vi "Create File Save Setup.vi"(8 "error in (no error)":errorcluster, 11 "Scan Data Process in":T1) -> (0 "error out":errorcluster, 3 "Scan Data Process out":T1)   [LabVIEW 2015, in "Exposure Process.lvlib"]
uses:
  Exposure Process.lvlib
  Control_Scan Data Process.ctl
  <vilib>/addons/PointValueMap/controls/PointMap.ctl
  Control_EXP Information.ctl
  Control_File Save Setup.ctl
  Control_Enable and Path.ctl
  Control_ICM Export Setting.ctl
  <vilib>/addons/PointValueMap/PointValueMap.lvlib
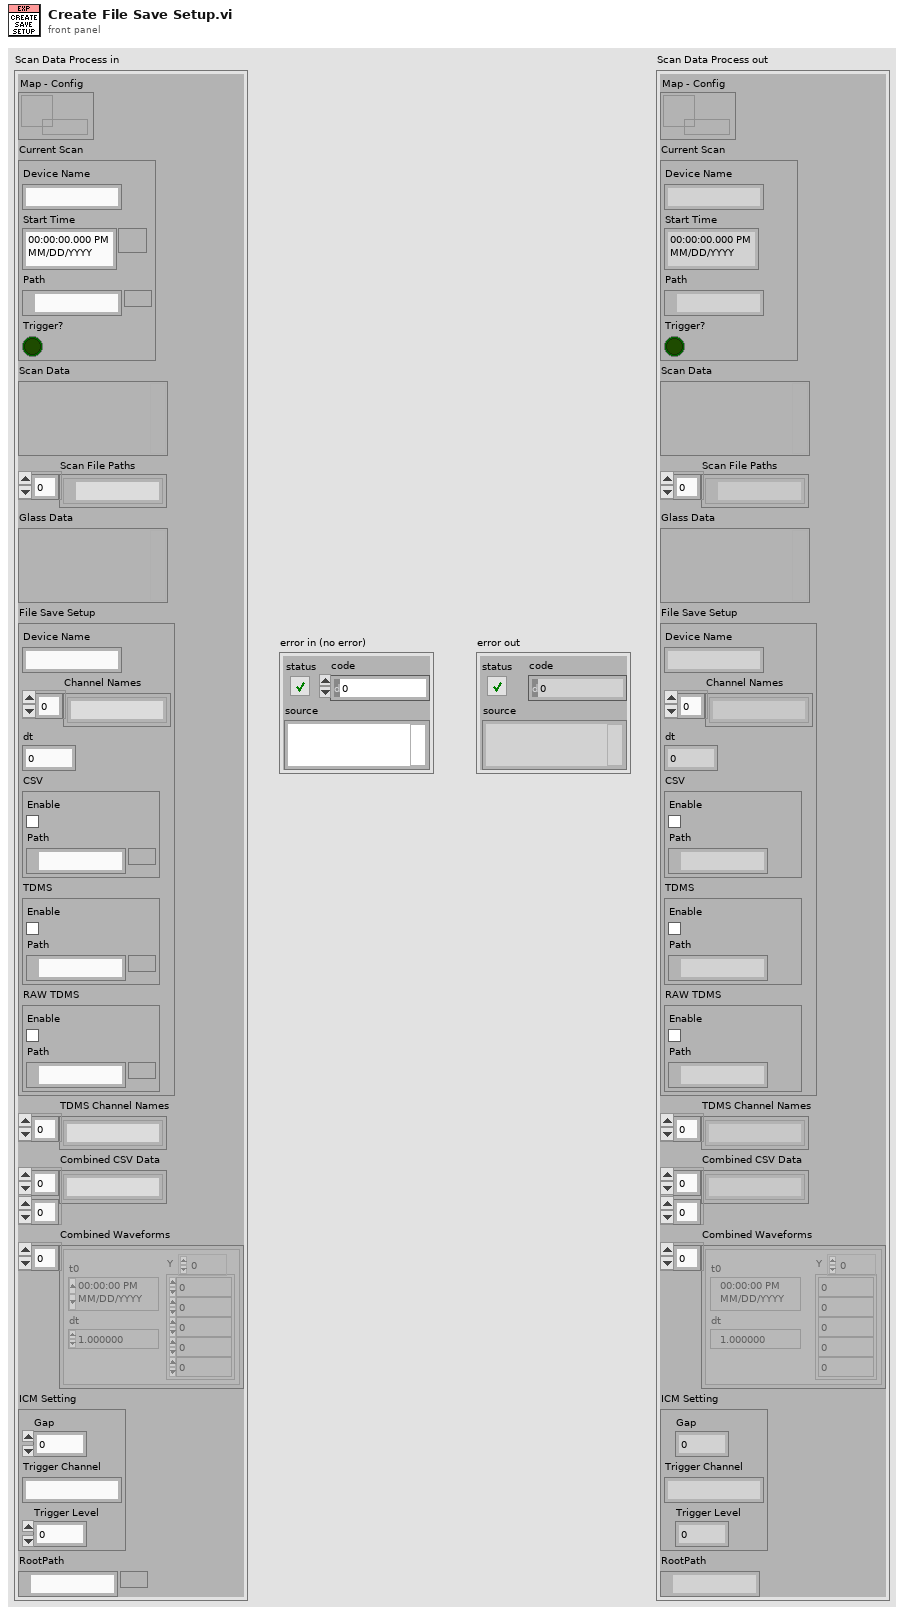
[diagram p1: front panel]
types:
  T1 = typedef "Exposure Process.lvlib/Control_Scan Data Process.ctl" = cluster{"Map - Config":T2, "Current Scan":T3, "Scan Data":variant, "Scan File Paths":path[], "Glass Data":variant, "File Save Setup":T4, "TDMS Channel Names":string[], "Combined CSV Data":string[][], "Combined Waveforms":waveform(dbl)[], "ICM Setting":T6, "RootPath":path}
  T2 = typedef "PointValueMap.lvlib/PointMap.ctl" = refnum<data-value>
  T3 = typedef "Exposure Process.lvlib/Control_EXP Information.ctl" = cluster{"Device Name":string, "Start Time":timestamp, "Path":path, "Trigger?":bool}
  T4 = typedef "Exposure Process.lvlib/Control_File Save Setup.ctl" = cluster{"Device Name":string, "Channel Names":string[], "dt":dbl, "CSV":T5, "TDMS":T5, "RAW TDMS":T5}
  T5 = typedef "Exposure Process.lvlib/Control_Enable and Path.ctl" = cluster{"Enable":bool, "Path":path}
  T6 = typedef "Exposure Process.lvlib/Control_ICM Export Setting.ctl" = cluster{"Gap":dbl, "Trigger Channel":string, "Trigger Level":dbl}
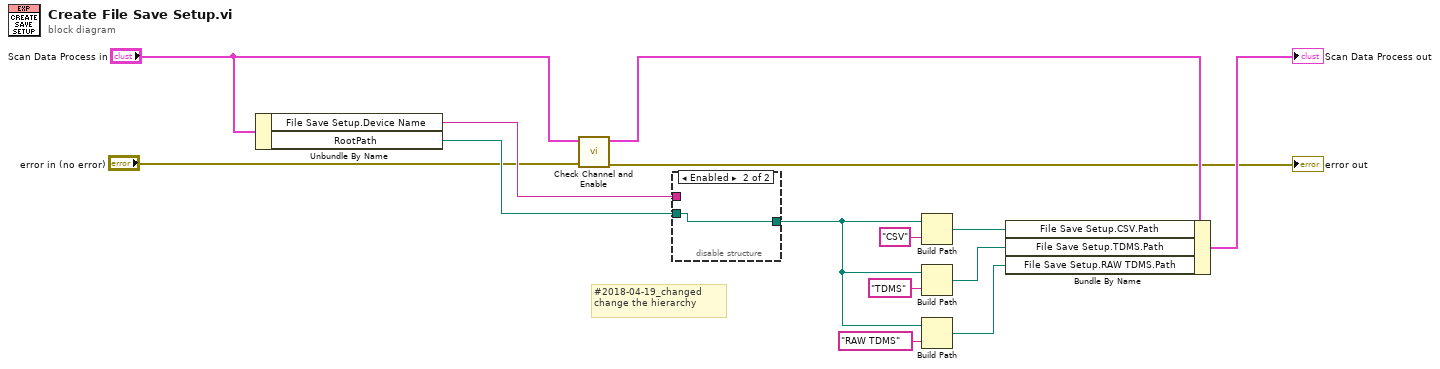
[diagram p0: block diagram]
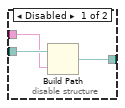
[diagram p2: hidden frame]
diagram:
  # "#2018-04-19_changed\nchange the hierarchy"
  n1 = Unbundle By Name("Scan Data Process in") -> ("File Save Setup.Device Name"=w6:string, "RootPath"=w2:path)
  n2 = call "Check Channel and Enable.vi"("error in (no error)"="error in (no error)", "Scan Data Process in"="Scan Data Process in") -> ("error out"=→"error out":errorcluster, "Scan Data Process out"=w4:T1)  [unwired: 8 in]
  n3 = disable-structure shown="Enabled" {
    disable-tunnel: [w17 w18] -> w8
    disable-tunnel: w2 -> [w16 w18]
    disable-tunnel: w6 -> [w15 _]
    frame Disabled {
      n4 = Build Path(base path=w16, name or relative path=w15) -> (appended path=w17:path)
    }
    frame Enabled {
    }
  }
  n5 = Build Path(base path=w8, name or relative path="CSV") -> (appended path=w11:path)
  n6 = Build Path(base path=w8, name or relative path="TDMS") -> (appended path=w10:path)
  n7 = Build Path(base path=w8, name or relative path="RAW TDMS") -> (appended path=w9:path)
  n8 = Bundle By Name(cluster=w4, "File Save Setup.CSV.Path"=w11, "File Save Setup.TDMS.Path"=w10, "File Save Setup.RAW TDMS.Path"=w9) -> (→"Scan Data Process out":T1)
